vi "SystemConfigSession.vi"(8 "error in":errorcluster) -> (0 "error out":errorcluster, 1 "Refnum out":refnum<k21>)   [LabVIEW 2020, in "hse-network.lvlib"]
doc: "(v0.2.1b; 2017-08-14 16:44)\n\n\n\n____\nHAMPEL SOFTWARE ENGINEERING v3.8.0 (2023-12-18 14:41)"
uses:
  hse-network.lvlib
  <vilib>/nisyscfg/nisyscfg.lvlib
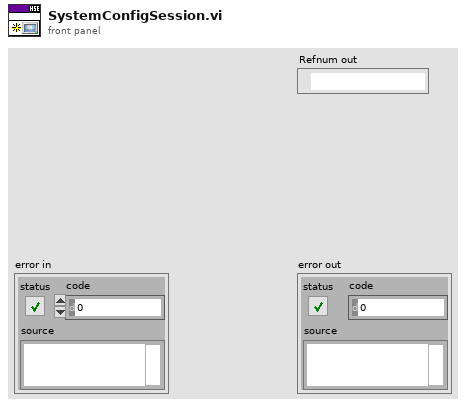
[diagram p1: front panel]
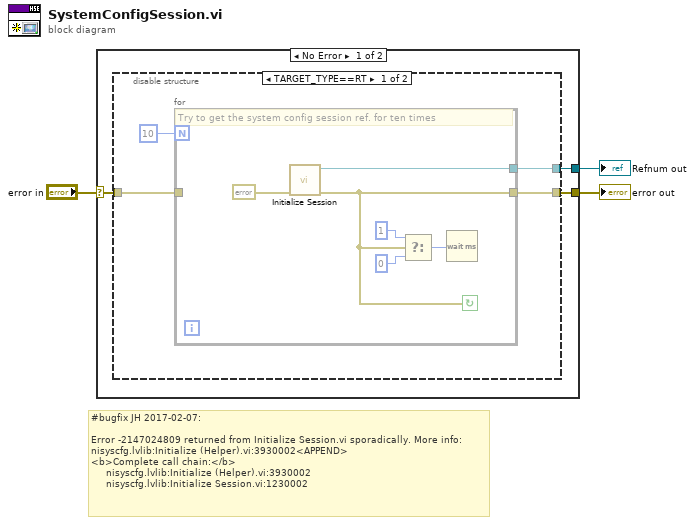
[diagram p0: block diagram]
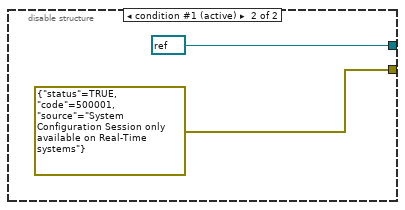
[diagram p2: hidden frame]
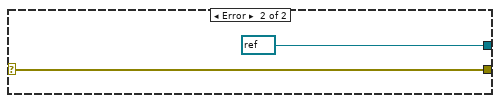
[diagram p3: hidden frame]
diagram:
  # "#bugfix JH 2017-02-07:\n\nError -2147024809 returned from Initialize Session.vi sporadically. More info:\nnisyscfg.lvlib:Initialize (Helper).vi:3930002<APPEND>\n<b>Complete call chain:</b>\n     nisyscfg.lvlib:Initialize (Helper).vi:3930002\n     nisyscfg.lvlib:Initialize Session.vi:1230002"
  n1 = case shown="No Error" "error in" {
    selector: "error in" -> [w4 w20]
    tunnel: [w6 refnum<k21> refnum ("Session out")] -> w3
    tunnel: [w5 w20] -> w2
    frame No Error {
      n2 = disable-structure shown="TARGET_TYPE==RT" {
        disable-tunnel: [w10 refnum<k21> refnum ("Refnum out")] -> w6
        disable-tunnel: [w9 errorcluster {"status"=TRUE, "code"=500001, "source"="System Configuration Session only available on Real-Time systems"} ("error in")] -> w5
        disable-tunnel: w4 -> [w8 _]
        frame condition #0 {
          n3 = for {
            N: 10 -> [_]
            tunnel: [w16] -> w10
            tunnel: w8 -> [_]
            tunnel: [w11] -> w9
            stop <- w11 continue-if-true
            # "Try to get the system config session ref. for ten times"
            n4 = call <vilib>:"Initialize Session.vi"("error in (no error)"=errorcluster {"status"=FALSE, "code"=0, "source"=""}) -> ("error out"=w11:errorcluster, "Session out"=w16:refnum<k21>)  [unwired: 9 in]
            n5 = Select(t=u32 1 ("milliseconds to wait"), s=w11, f=u32 0 ("milliseconds to wait")) -> (s? t:f=w12:u32)
            n6 = Wait (ms)(milliseconds to wait=w12) -> ()  [unwired: 1 out]
          }
        }
        frame condition #1 (active) {
        }
      }
    }
    frame Error {
    }
  }
  "Refnum out" <- w3
  "error out" <- w2
